vi "Finish.vi"   [LabVIEW 2013]
doc: "This VI is called just before exiting. It is expected to close I/O refnum, save collected data, etc."
uses:
  <vilib>/Rock Robotics/WPI/Joystick/WPI_JoystickGetSetRefNum.vi
  <vilib>/Rock Robotics/WPI/RobotDrive/WPI_RobotDriveGetSetRefNum.vi
types:
  T1 = typedef "WPI_RelayDevRef.ctl" = cluster{"DevStatus":errorcluster, "Relay Channel":T2, "Digital Module":T3, "Relay Direction":T4}
  T2 = typedef "FPGA_DIORelayChannel.ctl" = enum8{"Relay 1", "Relay 2", "Relay 3", "Relay 4", "Relay 5", "Relay 6", "Relay 7", "Relay 8", "Invalid"}
  T3 = typedef "FPGA_TypedefDigitalModule.ctl" = enum16{"Digital Module 1", "Digital Module 2"}
  T4 = typedef "WPI_RelayDirection.ctl" = enum16{"Both directions", "Forward only", "Reverse only"}
  T5 = typedef "WPI_DigitalInputDevRef.ctl" = cluster{"DevStatus":errorcluster, "DIO Channel":T6, "Digital Module":T3}
  T6 = typedef "FPGA_DIOChannel.ctl" = enum8{"DIO 1", "DIO 2", "DIO 3", "DIO 4", "DIO 5", "DIO 6", "DIO 7", "DIO 8", "DIO 9", "DIO 10", "DIO 11", "DIO 12", "DIO 13", "DIO 14", "Invalid"}
  T7 = typedef "WPI_JoystickDevRef.ctl" = cluster{"Device":T8}
  T8 = typedef "WPI_JoystickDeviceEnum.ctl" = enum16{"USB 1", "USB 2", "USB 3", "USB 4", "Kinect 1", "Kinect 2"}
  T9 = typedef "WPI_RobotDriveDevRef.ctl" = cluster{"DevStatus":errorcluster, "Motors[]":T10[], "Square Inputs":bool, "Max Output":dbl, "Isochronous":bool}
  T10 = typedef "WPI_MotorControlDeviceRef.ctl" = cluster{"DeviceStatus":errorcluster, "Type":enum16{"PWM", "CAN"}, "PWM":cluster{"Digital Module":T3, "PWM Channel":T11, "DeadBand":T12}, "CAN":cluster{"Device Number":u8, "Control Mode":T13, "Semaphore":T14, "Max Vout":dbl}, "Invert":bool, "TransformRef":T15, "InvTransformRef":T15}
  T11 = typedef "FPGA_DIOPWMChannel.ctl" = enum8{"PWM 1", "PWM 2", "PWM 3", "PWM 4", "PWM 5", "PWM 6", "PWM 7", "PWM 8", "PWM 9", "PWM 10", "Invalid"}
  T12 = typedef "WPI_PWMDeadband.ctl" = cluster{"Name":string, "maxPositivePwm":i32, "minPositivePwm":i32, "centerPwm":i32, "maxNegativePwm":i32, "minNegativePwm":i32, "angularRange":u16}
  T13 = typedef "WPI_CANJaguar_ControlMode.ctl" = enum8{"Percent VBus", "Current", "Speed", "Position", "Voltage"}
  T14 = typedef "Semaphore RefNum" = refnum<k1>
  T15 = typedef "WPI_PWMTransform_ConPane.ctl" = refnum<vi>
  T16 = typedef "WPI_CameraDevRef.ctl" = cluster{"Camera Address":string, "CameraStatus":errorcluster, "Acquire Image Notifier":refnum<notifier>}
  T17 = typedef "WPI_ServoDeviceRef.ctl" = cluster{"DeviceStatus":errorcluster, "Digital Module":T3, "PWM Channel":T11, "DeadBand":T12}
  T18 = typedef "WPI_EncoderDevRef.ctl" = cluster{"DevStatus":errorcluster, "EncoderIndex":T19, "CounterIndex":T20, "DistancePerCount":dbl, "Decoding Type":T21}
  T19 = typedef "FPGA_EncoderIdx.ctl" = enum8{"Enc 0", "Enc 1", "Enc 2", "Enc 3", "Invalid"}
  T20 = typedef "FPGA_CounterCtrSystemIndex.ctl" = enum8{"Ctr 0", "Ctr 1", "Ctr 2", "Ctr 3", "Ctr 4", "Ctr 5", "Ctr 6", "Ctr 7", "Invalid"}
  T21 = typedef "WPI_EncoderType.ctl" = enum16{"1x", "2x", "4x"}
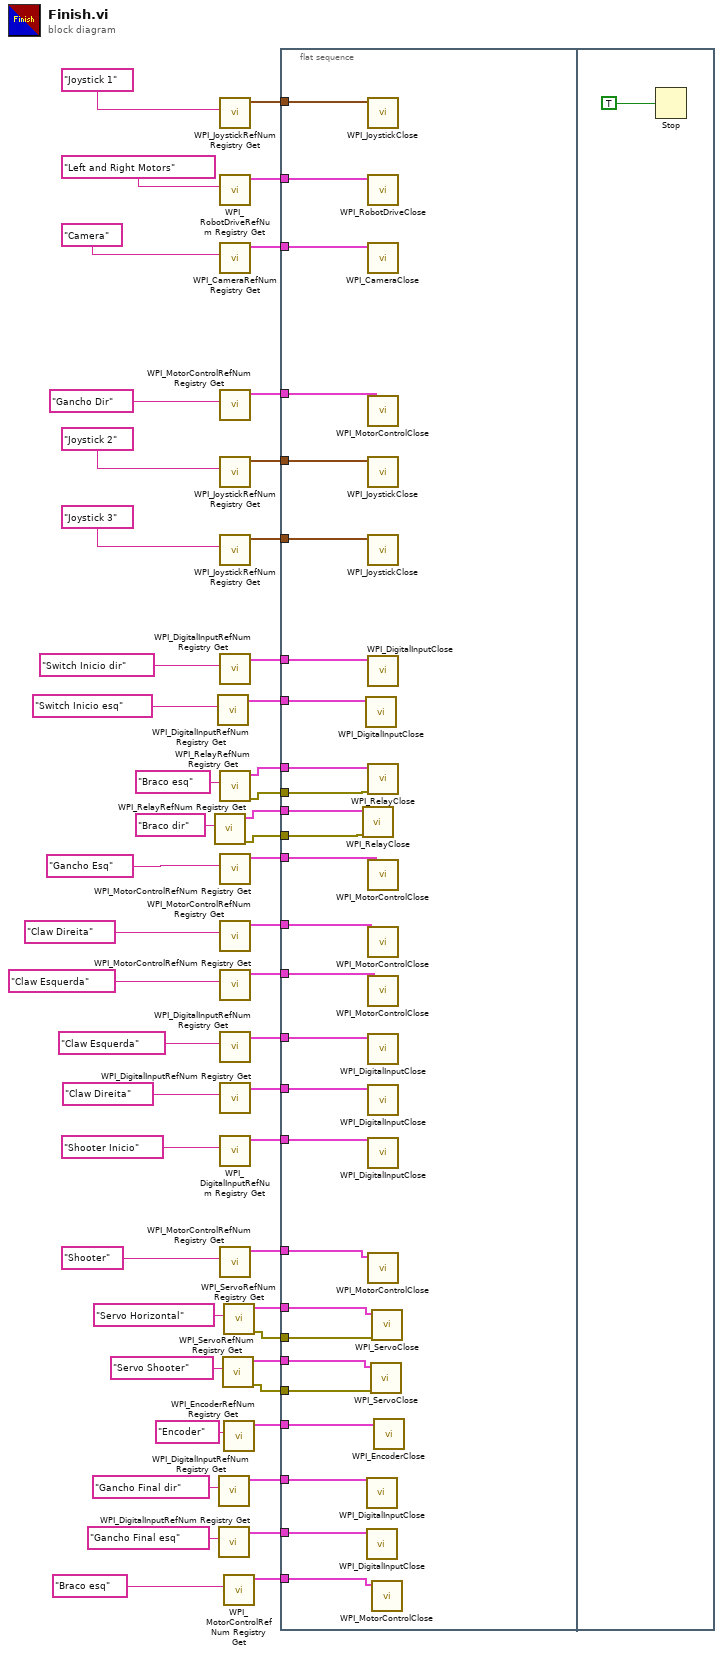
[diagram p0: block diagram]
diagram:
  n1 = call <vilib>:"WPI_RelayRefNum Registry Get.vi"("refnum name"="Braco dir") -> ("error out"=w4:errorcluster, "RelayDevRef"=w3:T1)  [unwired: 9 in]
  n2 = call <vilib>:"WPI_DigitalInputRefNum Registry Get.vi"("refnum name"="Switch Inicio esq") -> ("DigitalInputDevRef"=w10:T5)  [unwired: 9 in, 1 out]
  n3 = call <vilib>:"WPI_DigitalInputRefNum Registry Get.vi"("refnum name"="Gancho Final dir") -> ("DigitalInputDevRef"=w14:T5)  [unwired: 9 in, 1 out]
  n4 = call <vilib>:"WPI_DigitalInputRefNum Registry Get.vi"("refnum name"="Gancho Final esq") -> ("DigitalInputDevRef"=w13:T5)  [unwired: 9 in, 1 out]
  n5 = call <vilib>:"WPI_JoystickRefNum Registry Get.vi"("refnum name"="Joystick 1") -> ("JoystickDevRef"=w47:T7)  [unwired: 1 in, 9 out]
  n6 = call <vilib>:"WPI_RobotDriveRefNum Registry Get.vi"("refnum name"="Left and Right Motors") -> ("RobotDriveDevRef"=w48:T9)  [unwired: 1 in, 9 out]
  n7 = call <vilib>:"WPI_CameraRefNum Registry Get.vi"("refnum name"="Camera") -> ("CameraDevRef"=w46:T16)  [unwired: 1 in, 9 out]
  n8 = call <vilib>:"WPI_MotorControlRefNum Registry Get.vi"("refnum name"="Gancho Dir") -> ("MotorControlDevRef"=w44:T10)  [unwired: 9 in, 1 out]
  n9 = call <vilib>:"WPI_JoystickRefNum Registry Get.vi"("refnum name"="Joystick 2") -> ("JoystickDevRef"=w42:T7)  [unwired: 1 in, 9 out]
  n10 = call <vilib>:"WPI_JoystickRefNum Registry Get.vi"("refnum name"="Joystick 3") -> ("JoystickDevRef"=w39:T7)  [unwired: 1 in, 9 out]
  n11 = call <vilib>:"WPI_DigitalInputRefNum Registry Get.vi"("refnum name"="Switch Inicio dir") -> ("DigitalInputDevRef"=w37:T5)  [unwired: 9 in, 1 out]
  n12 = call <vilib>:"WPI_RelayRefNum Registry Get.vi"("refnum name"="Braco esq") -> ("error out"=w7:errorcluster, "RelayDevRef"=w8:T1)  [unwired: 9 in]
  n13 = call <vilib>:"WPI_MotorControlRefNum Registry Get.vi"("refnum name"="Gancho Esq") -> ("MotorControlDevRef"=w35:T10)  [unwired: 9 in, 1 out]
  n14 = call <vilib>:"WPI_MotorControlRefNum Registry Get.vi"("refnum name"="Claw Direita") -> ("MotorControlDevRef"=w33:T10)  [unwired: 9 in, 1 out]
  n15 = call <vilib>:"WPI_MotorControlRefNum Registry Get.vi"("refnum name"="Claw Esquerda") -> ("MotorControlDevRef"=w32:T10)  [unwired: 9 in, 1 out]
  n16 = call <vilib>:"WPI_DigitalInputRefNum Registry Get.vi"("refnum name"="Claw Esquerda") -> ("DigitalInputDevRef"=w27:T5)  [unwired: 9 in, 1 out]
  n17 = call <vilib>:"WPI_DigitalInputRefNum Registry Get.vi"("refnum name"="Claw Direita") -> ("DigitalInputDevRef"=w30:T5)  [unwired: 9 in, 1 out]
  n18 = call <vilib>:"WPI_DigitalInputRefNum Registry Get.vi"("refnum name"="Shooter Inicio") -> ("DigitalInputDevRef"=w25:T5)  [unwired: 9 in, 1 out]
  n19 = call <vilib>:"WPI_MotorControlRefNum Registry Get.vi"("refnum name"="Shooter") -> ("MotorControlDevRef"=w24:T10)  [unwired: 9 in, 1 out]
  n20 = call <vilib>:"WPI_ServoRefNum Registry Get.vi"("refnum name"="Servo Shooter") -> ("error out"=w18:errorcluster, "ServoDeviceRef"=w17:T17)  [unwired: 9 in]
  n21 = call <vilib>:"WPI_ServoRefNum Registry Get.vi"("refnum name"="Servo Horizontal") -> ("error out"=w21:errorcluster, "ServoDeviceRef"=w22:T17)  [unwired: 9 in]
  n22 = call <vilib>:"WPI_EncoderRefNum Registry Get.vi"("refnum name"="Encoder") -> ("EncoderDevRef"=w15:T18)  [unwired: 9 in, 1 out]
  n23 = call <vilib>:"WPI_MotorControlRefNum Registry Get.vi"("refnum name"="Braco esq") -> ("MotorControlDevRef"=w1:T10)  [unwired: 9 in, 1 out]
  n24 = flat-sequence {
    tunnel: w48 -> [w77]
    tunnel: w47 -> [w76]
    tunnel: w46 -> [w75]
    tunnel: w44 -> [w74]
    tunnel: w42 -> [w73]
    tunnel: w39 -> [w72]
    tunnel: w37 -> [w71]
    tunnel: w35 -> [w70]
    tunnel: w33 -> [w69]
    tunnel: w32 -> [w68]
    tunnel: w27 -> [w66]
    tunnel: w30 -> [w67]
    tunnel: w25 -> [w65]
    tunnel: w24 -> [w64]
    tunnel: w22 -> [w63]
    tunnel: w21 -> [w62]
    tunnel: w17 -> [w60]
    tunnel: w18 -> [w61]
    tunnel: w15 -> [w59]
    tunnel: w13 -> [w57]
    tunnel: w14 -> [w58]
    tunnel: w10 -> [w56]
    tunnel: w8 -> [w55]
    tunnel: w7 -> [w54]
    tunnel: w3 -> [w52]
    tunnel: w4 -> [w53]
    tunnel: w1 -> [w51]
    frame #0 {
      n25 = call <vilib>:"WPI_RelayClose.vi"("error in (no error)"=w53, "RelayDevRef"=w52) -> ()  [unwired: 9 in, 1 out]
      n26 = call <vilib>:"WPI_DigitalInputClose.vi"("DigitalInputDevRef"=w56) -> ()  [unwired: 10 in, 1 out]
      n27 = call <vilib>:"WPI_DigitalInputClose.vi"("DigitalInputDevRef"=w58) -> ()  [unwired: 10 in, 1 out]
      n28 = call <vilib>:"WPI_DigitalInputClose.vi"("DigitalInputDevRef"=w57) -> ()  [unwired: 10 in, 1 out]
      n29 = call <vilib>:"WPI_JoystickClose.vi"("JoystickDevRef"=w76) -> ()  [unwired: 11 out]
      n30 = call <vilib>:"WPI_RobotDriveClose.vi"("RobotDriveDevRef"=w77) -> ()  [unwired: 1 in, 10 out]
      n31 = call <vilib>:"WPI_CameraClose.vi"("CameraDevRef"=w75) -> ()  [unwired: 1 in, 10 out]
      n32 = call <vilib>:"WPI_MotorControlClose.vi"("MotorControlDevRef"=w74) -> ()  [unwired: 10 in, 1 out]
      n33 = call <vilib>:"WPI_JoystickClose.vi"("JoystickDevRef"=w73) -> ()  [unwired: 11 out]
      n34 = call <vilib>:"WPI_JoystickClose.vi"("JoystickDevRef"=w72) -> ()  [unwired: 11 out]
      n35 = call <vilib>:"WPI_DigitalInputClose.vi"("DigitalInputDevRef"=w71) -> ()  [unwired: 10 in, 1 out]
      n36 = call <vilib>:"WPI_RelayClose.vi"("error in (no error)"=w54, "RelayDevRef"=w55) -> ()  [unwired: 9 in, 1 out]
      n37 = call <vilib>:"WPI_MotorControlClose.vi"("MotorControlDevRef"=w70) -> ()  [unwired: 10 in, 1 out]
      n38 = call <vilib>:"WPI_MotorControlClose.vi"("MotorControlDevRef"=w69) -> ()  [unwired: 10 in, 1 out]
      n39 = call <vilib>:"WPI_MotorControlClose.vi"("MotorControlDevRef"=w68) -> ()  [unwired: 10 in, 1 out]
      n40 = call <vilib>:"WPI_DigitalInputClose.vi"("DigitalInputDevRef"=w66) -> ()  [unwired: 10 in, 1 out]
      n41 = call <vilib>:"WPI_DigitalInputClose.vi"("DigitalInputDevRef"=w67) -> ()  [unwired: 10 in, 1 out]
      n42 = call <vilib>:"WPI_DigitalInputClose.vi"("DigitalInputDevRef"=w65) -> ()  [unwired: 10 in, 1 out]
      n43 = call <vilib>:"WPI_MotorControlClose.vi"("MotorControlDevRef"=w64) -> ()  [unwired: 10 in, 1 out]
      n44 = call <vilib>:"WPI_ServoClose.vi"("error in (no error)"=w61, "MotorControlDevRef"=w60) -> ()  [unwired: 9 in, 1 out]
      n45 = call <vilib>:"WPI_ServoClose.vi"("error in (no error)"=w62, "MotorControlDevRef"=w63) -> ()  [unwired: 9 in, 1 out]
      n46 = call <vilib>:"WPI_MotorControlClose.vi"("MotorControlDevRef"=w51) -> ()  [unwired: 10 in, 1 out]
      n47 = call <vilib>:"WPI_EncoderClose.vi"("EncoderDevRef"=w59) -> ()  [unwired: 10 in, 1 out]
    }
    frame #1 {
      n48 = Stop(stop? (T)=TRUE ("Quit")) -> ()
    }
  }
